vi "Crash Test.vi"() -> ()   [LabVIEW 2019]
uses:
  gRPC - Example_1/Example_1_server/Example_1_server.lvlib
  gRPC - Example_2/Example_2_client/Example_2_client.lvlib
panel:
  out "error out":errorcluster
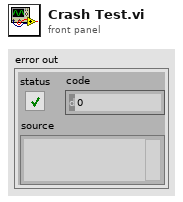
[diagram p1: front panel]
types:
  T1 = typedef "grpc-lvsupport-release.lvlib/grpcId.ctl" = u64
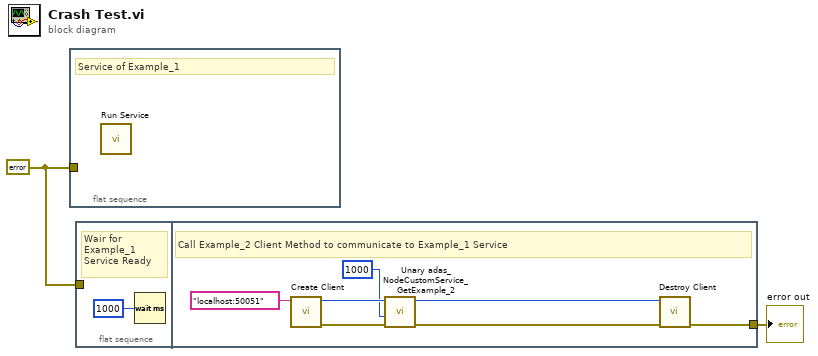
[diagram p0: block diagram]
diagram:
  w2 = errorcluster {"status"=FALSE, "code"=0, "source"=""} ("error in (no error)")
  n1 = flat-sequence {
    tunnel: w2 -> [_]
    frame #0 {
      # "Service of Example_1"
      n2 = call "Run Service.vi"() -> ()  [unwired: 12 in]
    }
  }
  n3 = flat-sequence {
    tunnel: w2 -> [_]
    tunnel: [w4] -> w1
    frame #0 {
      # "Wair for Example_1 Service Ready"
      n4 = Wait (ms)(milliseconds to wait=u32 1000) -> ()  [unwired: 1 out]
    }
    frame #1 {
      # "Call Example_2 Client Method to communicate to Example_1 Service"
      n5 = call "Create Client.vi"("address"="localhost:50051") -> ("error out"=w8:errorcluster, "gRPC ID Out"=w7:T1)  [unwired: 9 in]
      n6 = call "Unary adas_NodeCustomService_GetExample_2.vi"("error in"=w8, "timeout (ms)"=1000, "gRPC ID"=w7) -> ("error out"=w9:errorcluster, "gRPC ID out"=w10:T1)  [unwired: 6 in, 1 out]
      n7 = call "Destroy Client.vi"("error in"=w9, "gRPC ID"=w10) -> ("error out"=w4:errorcluster)  [unwired: 9 in]
    }
  }
  "error out" <- w1
